vi "Complex selector (waveform CDB).vi"(10 "Domain (mag)":T1, 11 "Waveform (CDB)":waveform(cdb)) -> (3 "Part (DBL)":waveform(dbl))   [LabVIEW 2020]
uses:
  Domain.ctl
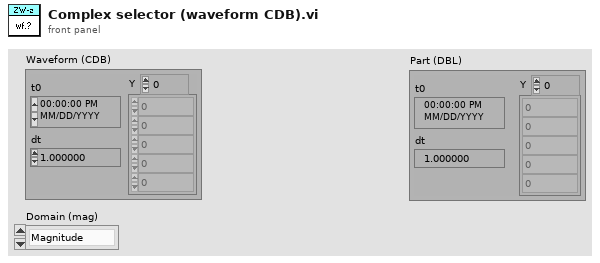
[diagram p1: front panel]
types:
  T1 = typedef "Domain.ctl" = enum16{"Magnitude", "Phase", "Phase unwrp", "Real", "Imaginary"}
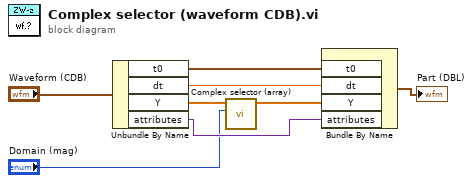
[diagram p0: block diagram]
diagram:
  n1 = Unbundle By Name("Waveform (CDB)") -> ("t0"=w4:timestamp, "dt"=w3:dbl, "Y"=w7:cdb[], "attributes"=w2:variant)
  n2 = call "Complex selector (array).vi"("Domain (mag)"="Domain (mag)", "Array (CDB)"=w7) -> ("Part (DBL)"=w6:dbl[])  [unwired: 9 in]
  n3 = Bundle By Name("t0"=w4, "dt"=w3, "Y"=w6, "attributes"=w2) -> (→"Part (DBL)":waveform(dbl))  [unwired: 1 in]
